vi "Write nodes.vi"(5 "nodes":i32[](array[numeric]), 9 "VI_AST in":refnum<class "VI_AST.lvclass">) -> (3 "VI_AST out":refnum<class "VI_AST.lvclass">)   [LabVIEW 2014, in "VI_AST.lvclass"]
uses:
  VI_AST.lvclass
  VI_AST.lvclass/VI_AST.ctl
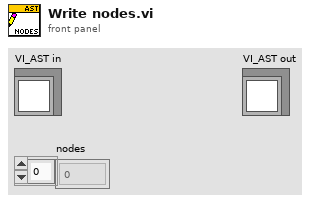
[diagram p1: front panel]
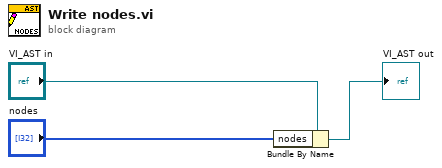
[diagram p0: block diagram]
diagram:
  n1 = Bundle By Name(cluster="VI_AST in", "nodes"="nodes") -> (→"VI_AST out":refnum<class "VI_AST.lvclass">)
